vi "Test10.vi"(5 "Peak":T2=enum."PCAN_USBBUS1", 7 "L2T":T1 caption="Limites de test pris en compte", 8 "errin":errorcluster, 9 "SN":string="0B5MEVA000CA1JC1M0000041", 10 "OCV":string) -> (0 "errout":errorcluster, 2 "chaîne concaténée":string, 4 "cluster de sortie":T3, 6 "v1":string)   [LabVIEW 2020]
uses:
  <userlib>/PCAN Basic/Controls/Channel.ctl
  Ctrl/L2T.ctl
  <userlib>/PCAN Basic/PCANBasic.lvlib
panel:
  # "Pre DCIR_____________________________________"
  # "intra DCIR_____________________________________"
  # "Post DCIR_____________________________________"
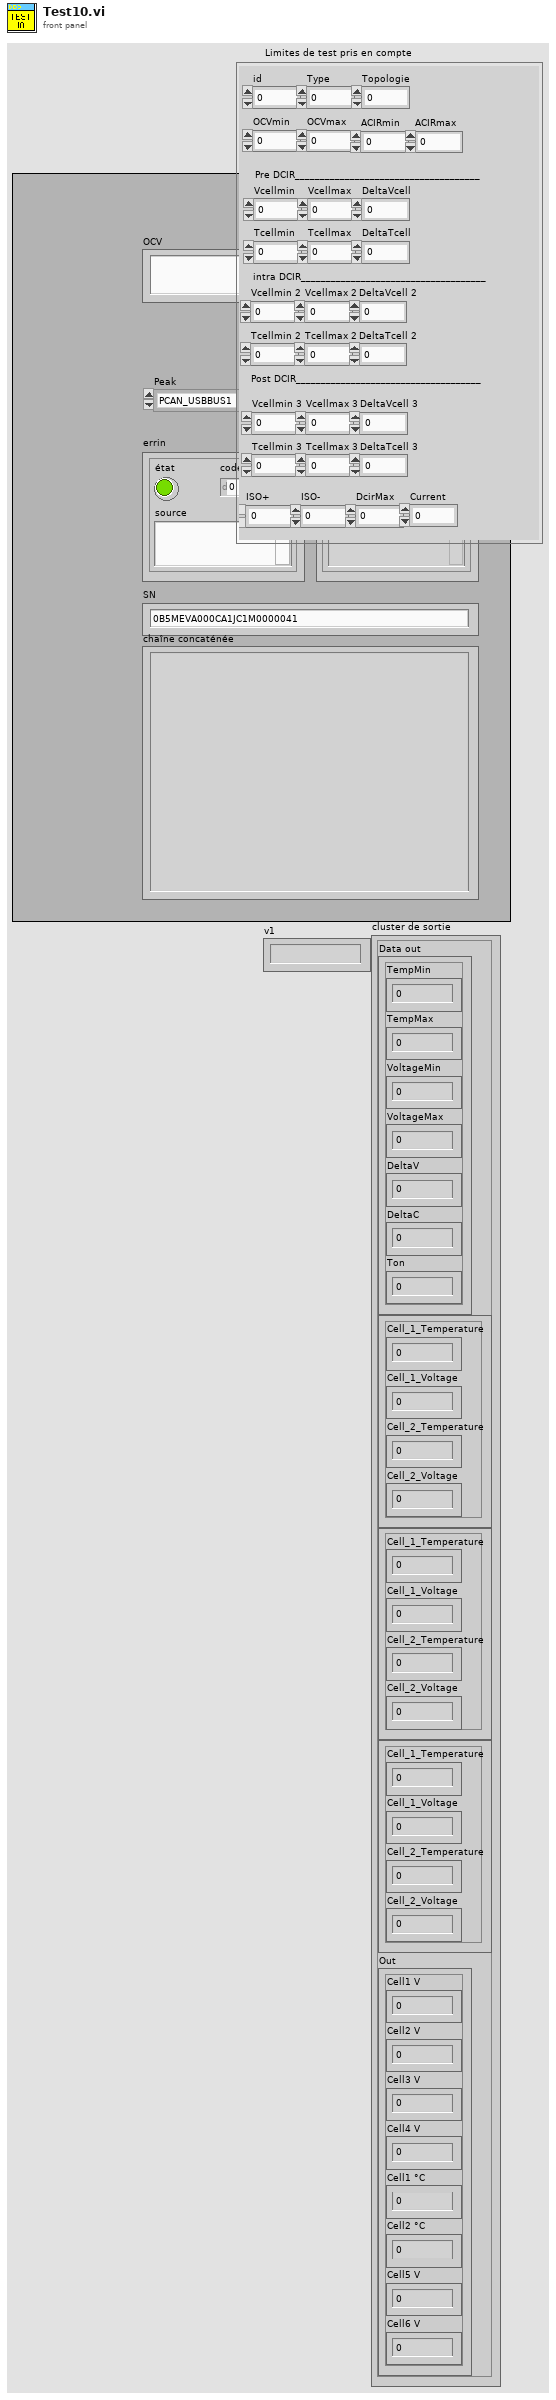
[diagram p1: front panel]
types:
  T1 = typedef "L2T.ctl" = cluster{"id":dbl, "Type":dbl, "OCVmin":dbl, "OCVmax":dbl, "ACIRmin":dbl, "ACIRmax":dbl, "Vcellmin":dbl, "Vcellmax":dbl, "DeltaVcell":dbl, "Tcellmin":dbl, "Tcellmax":dbl, "DeltaTcell":dbl, "ISO+":dbl, "ISO-":dbl, "DcirMax":dbl, "Current":dbl, "Topologie":dbl, "Vcellmin 2":dbl, "Vcellmax 2":dbl, "DeltaVcell 2":dbl, "Tcellmin 2":dbl, "Tcellmax 2":dbl, "DeltaTcell 2":dbl, "Vcellmin 3":dbl, "Vcellmax 3":dbl, "DeltaVcell 3":dbl, "Tcellmin 3":dbl, "Tcellmax 3":dbl, "DeltaTcell 3":dbl}
  T2 = typedef "PCANBasic.lvlib/Channel.ctl" = enum16{"PCAN_NONEBUS", "not used1", "not used2", "not used3", "not used4", "not used5", "not used6", "not used7", "not used8", "not used9", "not used10", "not used11", "not used12", "not used13", "not used14", "not used15", "not used16", "not used17", "not used18", "not used19", "not used20", "not used21", "not used22", "not used23", "not used24", "not used25", "not used26", "not used27", "not used28", "not used29", "not used30", "not used31", "not used32", "PCAN_ISABUS1", "PCAN_ISABUS2", "PCAN_ISABUS3", "PCAN_ISABUS4", "PCAN_ISABUS5", "PCAN_ISABUS6", "PCAN_ISABUS7", "PCAN_ISABUS8", "not used41", "not used42", "not used43", "not used44", "not used45", "not used46", "not used47", "not used48", "PCAN_DNGBUS1", "not used50", "not used51", "not used52", "not used53", "not used54", "not used55", "not used56", "not used57", "not used58", "not used59", "not used60", "not used61", "not used62", "not used63", "not used64", "PCAN_PCIBUS1", "PCAN_PCIBUS2", "PCAN_PCIBUS3", "PCAN_PCIBUS4", "PCAN_PCIBUS5", "PCAN_PCIBUS6", "PCAN_PCIBUS7", "PCAN_PCIBUS8", "not used73", "not used74", "not used75", "not used76", "not used77", "not used78", "not used79", "not used80", "PCAN_USBBUS1", "PCAN_USBBUS2", "PCAN_USBBUS3", "PCAN_USBBUS4", "PCAN_USBBUS5", "PCAN_USBBUS6", "PCAN_USBBUS7", "PCAN_USBBUS8", "Not used89", "Not used90", "Not used91", "Not used92", "Not used93", "Not used94", "Not used95", "Not used96", "PCAN_PCCBUS1", "PCAN_PCCBUS2"}
  T3 = cluster{"Data out":cluster{"TempMin":sgl, "TempMax":sgl, "VoltageMin":sgl, "VoltageMax":sgl, "DeltaV":sgl, "DeltaC":sgl, "Ton":sgl}, "Cluster":cluster{"Cell_1_Temperature":sgl, "Cell_1_Voltage":sgl, "Cell_2_Temperature":sgl, "Cell_2_Voltage":sgl}, "Cluster":cluster{"Cell_1_Temperature":sgl, "Cell_1_Voltage":sgl, "Cell_2_Temperature":sgl, "Cell_2_Voltage":sgl}, "Cluster":cluster{"Cell_1_Temperature":sgl, "Cell_1_Voltage":sgl, "Cell_2_Temperature":sgl, "Cell_2_Voltage":sgl}, "Out":cluster{"Cell1 V":sgl, "Cell2 V":sgl, "Cell3 V":sgl, "Cell4 V":sgl, "Cell1 °C":sgl, "Cell2 °C":sgl, "Cell5 V":sgl, "Cell6 V":sgl}}
  T4 = cluster{"Cell1 V":sgl, "Cell2 V":sgl, "Cell3 V":sgl, "Cell4 V":sgl, "Cell1 °C":sgl, "Cell2 °C":sgl, "Cell5 V":sgl, "Cell6 V":sgl}
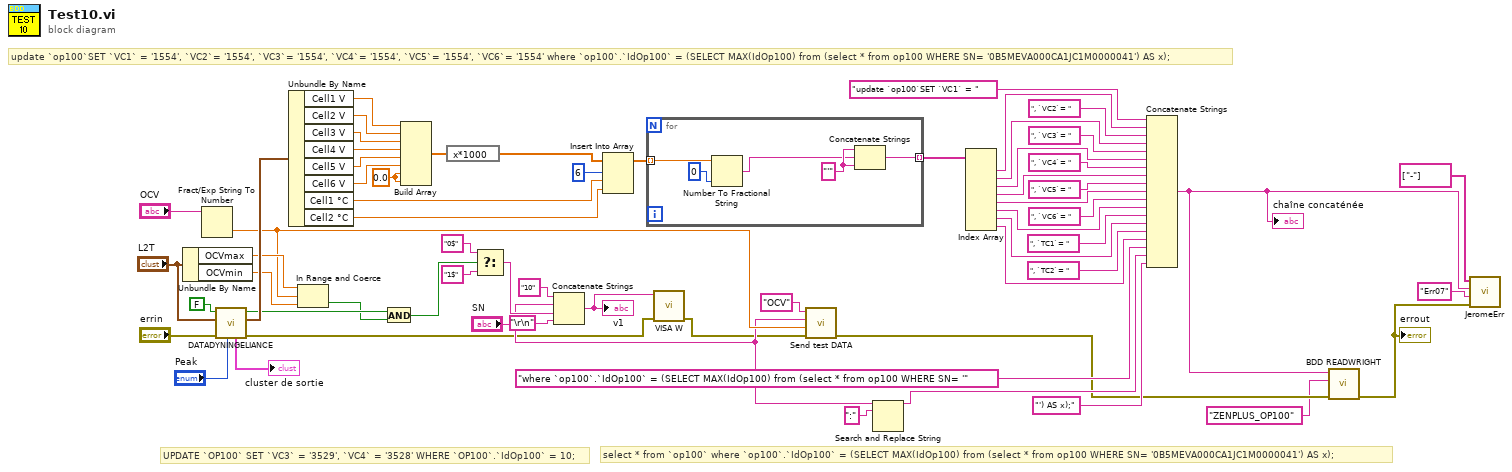
[diagram p0: block diagram]
diagram:
  w48 = sgl 0.0 ("élément")
  # "select * from `op100` where `op100`.`IdOp100` = (SELECT MAX(IdOp100) from (select * from op100 WHERE SN= '0B5MEVA000CA1JC1M0000041') AS x);"
  # "update `op100`SET `VC1` = '1554', `VC2`= '1554', `VC3`= '1554', `VC4`= '1554', `VC5`= '1554', `VC6`= '1554' where `op100`.`IdOp100` = (SELECT MAX(IdOp100) from (select * from op100 WHERE SN= '0B5MEVA000CA1JC1M0000041') AS x);"
  # "UPDATE `OP100` SET `VC3` = '3529', `VC4` = '3528' WHERE `OP100`.`IdOp100` = 10;"
  n1 = Unbundle By Name("L2T") -> ("OCVmax"=w25:dbl, "OCVmin"=w24:dbl)
  n2 = Fract/Exp String To Number ("Chaîne Fract/Exp en nombre")(string="OCV") -> (number=w14:dbl)  [unwired: 3 in, 1 out]
  n3 = call "DATADYNINGELIANCE.vi"("Channel"="Peak", "errin"="errin", "L2T"="L2T", "3P4S"=FALSE) -> ("errout"=w8:errorcluster, "Out"=w51:T4, "test OK?"=w21:bool, "cluster de sortie"=→"cluster de sortie":T3)  [unwired: 3 in, 1 out]
  n4 = Unbundle By Name(w51) -> ("Cell1 V"=w52:sgl, "Cell2 V"=w53:sgl, "Cell3 V"=w54:sgl, "Cell4 V"=w55:sgl, "Cell5 V"=w56:sgl, "Cell6 V"=w57:sgl, "Cell1 °C"=w61:sgl, "Cell2 °C"=w62:sgl)
  n5 = In Range and Coerce(upper limit=w25, x=w14, lower limit=w24) -> (In Range?=w20:bool)  [unwired: 1 out]
  n6 = And(x=w21, y=w20) -> (x .and. y?=w19:bool)
  n7 = Build Array(w52, w53, w54, w55, w56, w57, w48, w48) -> (w58:sgl[])
  n8 = expression code="x*1000"(w58) -> (w59:sgl[])
  n9 = Select(t="0$" ("chaîne"), s=w19, f="1$" ("chaîne")) -> (s? t:f=w17:string)
  n10 = Concatenate Strings("10" ("chaîne"), "SN", w17, "\r\n") -> (w6:string)
  "v1" <- w6
  n11 = Insert Into Array(array=w59, index=6 ("indice"), new element #1=w61, new element #2=w62) -> (w63:sgl[])
  n12 = for {
    tunnel: w63 -> [w68] mode=indexing
    tunnel: [w65] -> w42 mode=indexing
    w66 = "'" ("chaîne")
    n13 = Number To Fractional String ("Nombre en chaîne fractionnaire")(number=w68, precision (6)=i16 0 ("précision (6)")) -> (F-format string=w64:string)  [unwired: 2 in]
    n14 = Concatenate Strings(w66, w64, w66) -> (w65:string)
  }
  n15 = call "VISA W.vi"("errin"=w8, "Chaîne"=w6) -> ("errout"=w7:errorcluster)  [unwired: 9 in]
  n16 = call "Send test DATA.vi"("errin"=w7, "Value"=w14, "SN"="SN", "test"="OCV") -> ("error out"=w4:errorcluster)  [unwired: 7 in]
  n17 = Search and Replace String ("Rechercher et remplacer une chaîne")(input string="SN", search string=":" ("chaîne recherchée")) -> (result string=w44:string)  [unwired: 6 in, 3 out]
  n18 = Index Array(array=w42) -> (element #1=w41:string, element #2=w39:string, element #3=w37:string, element #4=w35:string, element #5=w33:string, element #6=w31:string, element #7=w30:string, element #8=w27:string)  [unwired: 8 in]
  n19 = Concatenate Strings("update `op100`SET `VC1` = " ("chaîne"), w41, ", `VC2`= " ("chaîne"), w39, ", `VC3`= " ("chaîne"), w37, ", `VC4`= " ("chaîne"), w35, ", `VC5`= " ("chaîne"), w33, ", `VC6`= " ("chaîne"), w31, ", `TC1`= " ("chaîne"), w30, ", `TC2`= " ("chaîne"), w27, "where `op100`.`IdOp100` = (SELECT MAX(IdOp100) from (select * from op100 WHERE SN= '" ("chaîne"), w44, "') AS x);" ("chaîne")) -> (w2:string)
  "chaîne concaténée" <- w2
  n20 = call <userlib>:"BDD READWRIGHT.vi"("errin"=w4, "DSN name"="ZENPLUS_OP100", "Instruction"=w2) -> ("error out"=w1:errorcluster)  [unwired: 7 in, 1 out]
  "errout" <- w1
  n21 = call "JeromeErr.vi"("Errin"=w1, "CodeERR"="Err07", "RequetteSQL"=w2, "RetourSQL"=string[] ["-"]) -> ()  [unwired: 8 in]
